vi "Sylvester Equations.vi"   [LabVIEW 2017, in "NI_AALPro.lvlib"]
doc: "Solves the Sylvester matrix equation. The data types you wire to the <B>A</B>, <B>B</B>, and <B>C</B> inputs determine the polymorphic instance to use."
uses:
  NI_AALPro.lvlib
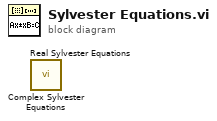
[diagram p0: block diagram]
diagram:
  n1 = call "Complex Sylvester Equations.vi"() -> ()  [unwired: 8 in, 4 out]
  n2 = call "Real Sylvester Equations.vi"() -> ()  [unwired: 8 in, 4 out]
